vi "lockin.SMO.vi"() -> ()   [LabVIEW 2016]
uses:
  <vilib>/JKI/JKI SMO/SMO/Typedefs/SMOState --Enum.ctl
  DAQ/Typedefs/DAQ.Config.ctl
  DAQ/Typedefs/PrivateEvents--DAQ.AI.Channels.ctl
  DAQ/Typedefs/DAQType.ctl
  DAQ/Typedefs/SamplingInfo.ctl
  DAQ/Typedefs/SamplingMode.ctl
  DAQmx/DAQmx.lvclass
  C:/user/patrick/hg/lockin.SMO/lvsrc/DAQ/DAQ.lvclass
  DAQ/DAQ.lvclass
  C:/Program Files (x86)/National Instruments/LabVIEW 2016/vi.lib/JKI/JKI SMO/SMO/SMO.lvclass
  <vilib>/JKI/JKI SMO/SMO/SMO.lvclass
panel:
  in  "Configuration":T1={"Channels"="", "DAQType"=enum."AI", "minimum value"=-5.0, "maximum value"=5.0, "sampling info"={"Fs"=0.0, "#s"=0.0}, "SamplingMode"=enum."Continuous"} {"maximum value" format="%0.2f"; "minimum value" format="%0.2f"}
  in  "Simulate?":bool
  out "Write":T6(graph)
  out "Read":T7(graph)
  out "SMO State":T8
  out "error out":errorcluster
  in  "Stop":bool
  # "Lockin SMO Test Launcher"
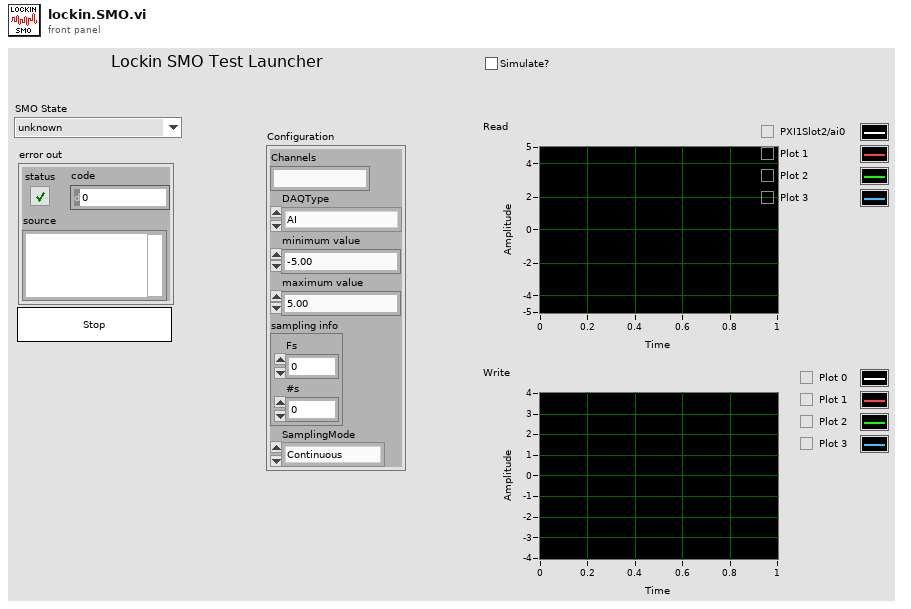
[diagram p1: front panel]
types:
  T1 = typedef "DAQ.lvclass/DAQ.Config.ctl" = cluster{"Channels":T2, "DAQType":T3, "minimum value":dbl, "maximum value":dbl, "sampling info":T4, "SamplingMode":T5}
  T2 = typedef "PrivateEvents--DAQ.AI.Channels.ctl" = string
  T3 = typedef "DAQ.lvclass/DAQType.ctl" = enum16{"AI", "AO"}
  T4 = typedef "DAQ.lvclass/SamplingInfo.ctl" = cluster{"Fs":dbl, "#s":dbl}
  T5 = typedef "DAQ.lvclass/SamplingMode.ctl" = enum16{"Continuous", "Finite"}
  T6 = typedef "DAQ.lvclass/PublicEvents--DAQ.Write.ctl" = waveform(dbl)[]
  T7 = typedef "DAQ.lvclass/PublicEvents--DAQ.Read.ctl" = waveform(dbl)[]
  T8 = typedef "SMO.lvclass/SMOState --Enum.ctl" = enum16{"unknown", "Created", "Started", "Stopped"}
  T9 = typedef "SMO.lvclass/Public Events.ctl" = cluster{"Error":refnum<user-event>, "State":refnum<user-event>, "Reserve State":refnum<user-event>}
  T10 = typedef "DAQ.lvclass/PublicEvents--Cluster.ctl" = cluster{"Read":refnum<user-event>, "Write":refnum<user-event>}
  T11 = cluster{"Event Registration Refnum":refnum<event-registration>}
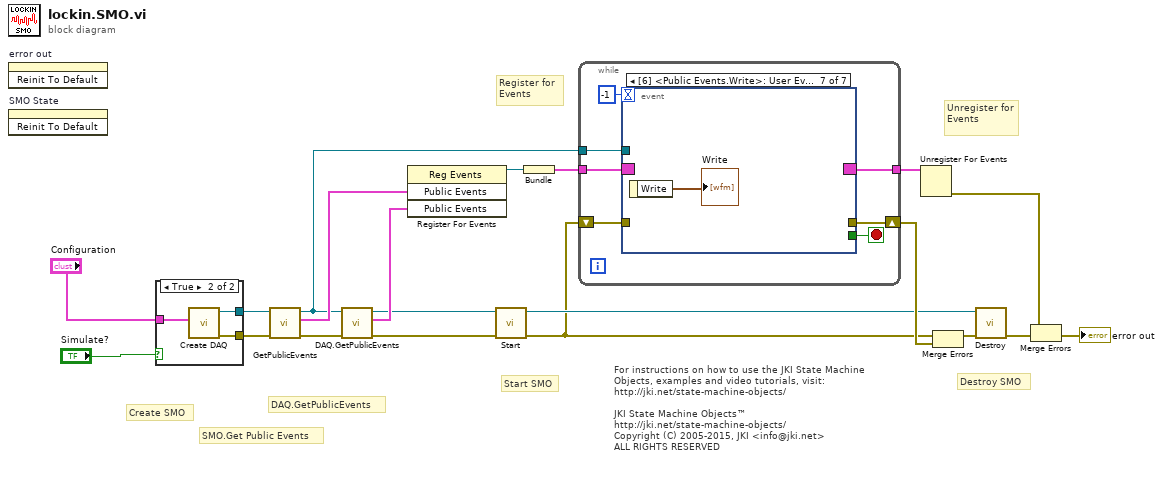
[diagram p0: block diagram]
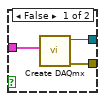
[diagram p2: hidden frame]
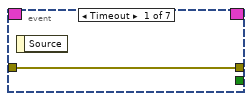
[diagram p3: hidden frame]
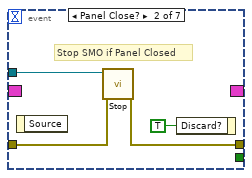
[diagram p4: hidden frame]
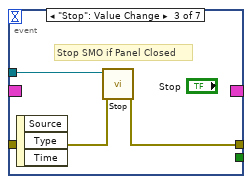
[diagram p5: hidden frame]
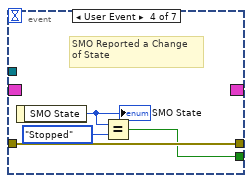
[diagram p6: hidden frame]
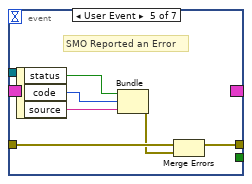
[diagram p7: hidden frame]
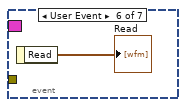
[diagram p8: hidden frame]
diagram:
  # "DAQ.GetPublicEvents"
  # "For instructions on how to use the JKI State Machine Objects, examples and video tutorials, visit:\nhttp://jki.net/state-machine-objects/\n\nJKI State Machine Objects™\nhttp://jki.net/state-machine-objects/\nCopyright (C) 2005-2015, JKI <info@jki.net>\nALL RIGHTS RESERVED"
  # "SMO.Get Public Events"
  # "Start SMO"
  # "Destroy SMO"
  # "Create SMO"
  # "Unregister for Events"
  # "Register for Events"
  n1 = invoke on="error out" class="Clust (strict)" method="Reinit To Default"() -> ()  [unwired: 3 in, 3 out]
  n2 = invoke on="SMO State" class="Enum (strict)" method="Reinit To Default"() -> ()  [unwired: 3 in, 3 out]
  n3 = case shown="True" "Simulate?" {
    tunnel: [w22 w26] -> w6
    tunnel: [w23 w25] -> w5
    tunnel: "Configuration" -> [w21 w24]
    frame False {
      n4 = call "Create DAQmx.vi"("Configuration"=w21) -> ("error out"=w22:errorcluster, "DAQmx out"=w23:refnum<class "DAQmx.lvclass">)  [unwired: 9 in]
    }
    frame True {
      n5 = call "Create DAQ.vi"("Configuration"=w24) -> ("error out"=w26:errorcluster, "DAQ out"=w25:refnum<class "DAQ.lvclass">)  [unwired: 9 in]
    }
  }
  n6 = call <vilib>:"GetPublicEvents.vi"("error in (no error)"=w6, "SMO"=w5) -> ("error out"=w9:errorcluster, "Public Events"=w12:T9, "SMO out"=w10:refnum<class "DAQ.lvclass">)  [unwired: 7 in]
  n7 = call "DAQ.GetPublicEvents.vi"("error in (no error)"=w9, "DAQ"=w10) -> ("error out"=w3:errorcluster, "Public Events"=w8:T10, "DAQ out"=w4:refnum<class "DAQ.lvclass">)  [unwired: 7 in]
  n8 = register-events(w12, w8) -> (reference out=w11:refnum<event-registration>)  [unwired: 2 in, 1 out]
  n9 = call <vilib>:"Start.vi"("error in (no error)"=w3, "SMO"=w4) -> ("error out"=w7:errorcluster, "SMO out"=w13:refnum<class "DAQ.lvclass">)  [unwired: 8 in]
  n10 = Bundle("Event Registration Refnum"=w11) -> (w19:T11)  [unwired: 1 in]
  n11 = while {
    shift-right: [w32] -> w18
    shift-left: w7 -> [w31]
    tunnel: w19 -> [w30]
    tunnel: [w29] -> w20
    tunnel: w10 -> [w28]
    stop <- w33 stop-if-true
    n12 = event shown="[6] <Public Events.Write>: User Event" {
      selector: w30 -> [_ _ _ _ _ _ _]
      dyn-events: [_ _ _ _ _ _ _] -> w29
      timeout: -1 -> [_ _ _ _ _ _ _]
      tunnel: [_ _ _ w42 _ _ _] -> w33
      tunnel: w28 -> [_ w38 w41 _ _ _ _]
      tunnel: [w34 w37 w40 w45 w49 _ _] -> w32
      tunnel: w31 -> [w34 w36 w39 w45 w47 _ _]
      event Timeout {
        n13 = event-data() -> ()  [unwired: 1 in, 1 out]
      }
      event Panel Close? {
        # "Stop SMO if Panel Closed"
        n14 = event-data() -> ()  [unwired: 1 in, 1 out]
        n15 = call <vilib>:"Stop.vi"("error in (no error)"=w36, "SMO"=w38) -> ("error out"=w37:errorcluster)  [unwired: 8 in, 1 out]
        n16 = event-data("Discard?"=TRUE ("OK")) -> ()  [unwired: 1 in, 1 out]
      }
      event "Stop": Value Change {
        # "Stop SMO if Panel Closed"
        n17 = event-data() -> ()  [unwired: 1 in, 3 out]
        n18 = call <vilib>:"Stop.vi"("error in (no error)"=w39, "SMO"=w41) -> ("error out"=w40:errorcluster)  [unwired: 8 in, 1 out]
      }
      event User Event {
        # "SMO Reported a Change\nof State"
        n19 = event-data() -> ("SMO State"=w44:T8)  [unwired: 1 in]
        "SMO State" <- w44
        n20 = Equal?(x=w44, y=SMOState_--Enum."Stopped") -> (x = y?=w42:bool)
      }
      event User Event {
        # "SMO Reported an Error"
        n21 = event-data() -> ("status"=w48:bool, "code"=w51:i32, "source"=w50:string)  [unwired: 1 in]
        n22 = Bundle("status"=w48, "code"=w51, "source"=w50) -> (w46:errorcluster)  [unwired: 1 in]
        n23 = Merge Errors(w47, w46) -> (w49:errorcluster)
      }
      event User Event {
        n24 = event-data() -> ("Read"=→"Read":T7)  [unwired: 1 in]
      }
      event User Event {
        n25 = event-data() -> ("Write"=→"Write":T6)  [unwired: 1 in]
      }
    }
  }
  n26 = Unregister For Events(event registration refnum=w20) -> (error out=w17:errorcluster)  [unwired: 1 in]
  n27 = Merge Errors(w7, w18) -> (w14:errorcluster)
  n28 = call <vilib>:"Destroy.vi"("error in (no error)"=w14, "SMO"=w13) -> ("error out"=w15:errorcluster)  [unwired: 9 in]
  n29 = Merge Errors(w17, w15) -> (→"error out":errorcluster)
